vi "Strings and Values.vi"(8 "error in (no error)":errorcluster, 11 "Dynamic Values in":refnum<class "Dynamic Values.lvclass">) -> (0 "error out":errorcluster, 2 "Strings And Values []":T1, 3 "Dynamic Values out":refnum<class "Dynamic Values.lvclass">)   [LabVIEW 2020, in "Dynamic Combobox.lvlib" / "Dynamic Values.lvclass"]
uses:
  Dynamic Values.lvclass
  <vilib>/Utility/miscctls.llb/LVComboBoxStrsAndValuesArrayTypeDef.ctl
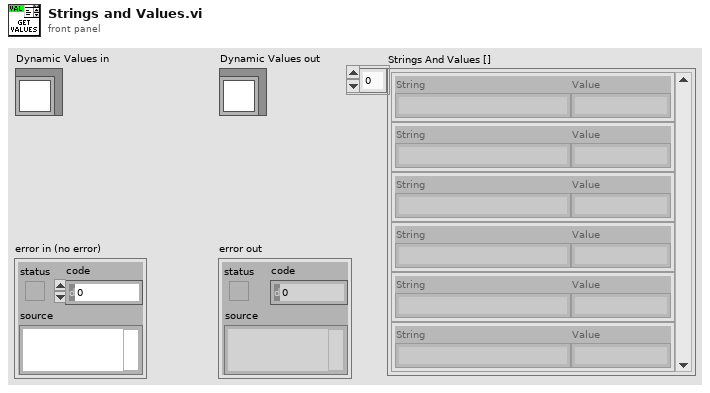
[diagram p1: front panel]
types:
  T1 = typedef "LVComboBoxStrsAndValuesArrayTypeDef.ctl" = cluster{"String":string, "Value":string}[]
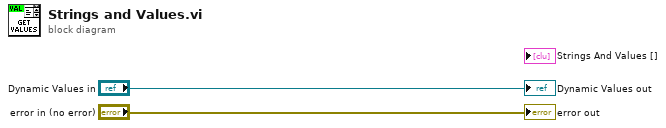
[diagram p0: block diagram]
diagram:
  "error out" <- "error in (no error)"
  "Dynamic Values out" <- "Dynamic Values in"
